vi "Database.Reload.vi"(7 "Idx":i32, 8 "error in":errorcluster, 11 "Data in":T1) -> (0 "error out":errorcluster, 3 "Data out":T1)   [LabVIEW 2016]
doc: "Connect to database\n\nWabco 2017 All right reserved\nAuthor: maciej.szupienko@wabco-auto.com"
uses:
  Database.Global.vi
  Cache/Cache.SystemID.Fglb.Action.ctl
  Cache/Cache.TestSteps.Fglb.Action.ctl
  ProdaNG/Controls/ProdaNG.TestStepParam.ctl
  ProdaNG/Controls/ProdaNG.TestValue.ctl
  ProdaNG/Controls/ProdaNG.TestStep.ctl
  Cache/Cache.TestSteps.Fglb.ResultData.ctl
  ProdaNG/Controls/ProdaNG.TestValueResult.ctl
  ProdaNG/Controls/ProdaNG.TestStepResult.ctl
  ProdaNG/Controls/ProdaNG.ProcessStepResult.ctl
  ProdaNG/Controls/ProdaNG.ProcessResult.ctl
  ProdaNG/Controls/ProdaNG.ProcessStepParam.ctl
  Cache/Cache.TestSteps.Fglb.TestData.ctl
  ProdaNG/Controls/ProdaNG.Unit.ctl
  ProdaNG/Controls/ProdaNG.Process.ctl
  ProdaNG/Controls/ProdaNG.ProcessStep.ctl
  Database.Data.Status.ctl
  Database.Data.Sets.ctl
  Database.Data.ctl
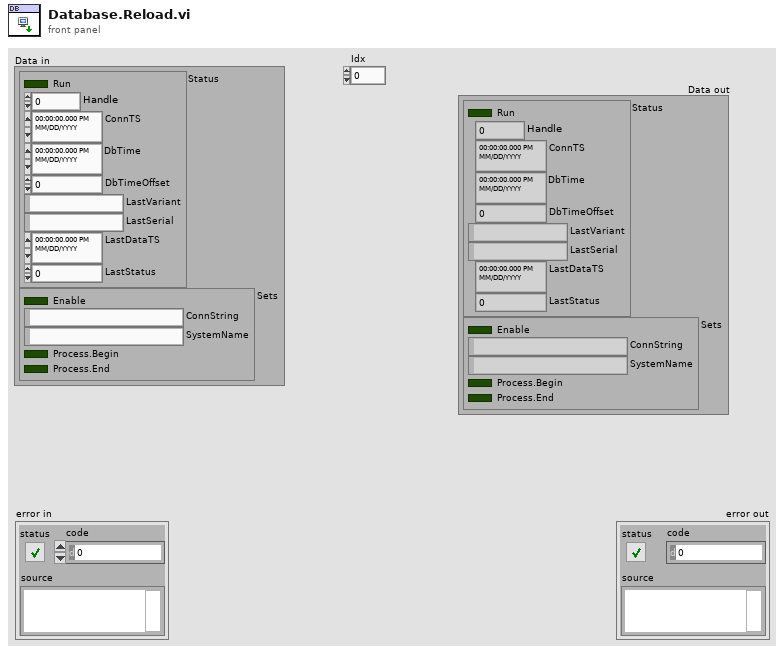
[diagram p1: front panel]
types:
  T1 = typedef "Database.Data.ctl" = cluster{"Status":T2, "Sets":T3}
  T2 = typedef "Database.Data.Status.ctl" = cluster{"Run":bool, "Handle":i32, "ConnTS":timestamp, "DbTime":timestamp, "DbTimeOffset":dbl, "LastVariant":string, "LastSerial":string, "LastDataTS":timestamp, "LastStatus":i32}
  T3 = typedef "Database.Data.Sets.ctl" = cluster{"Enable":bool, "ConnString":string, "SystemName":string, "Process.Begin":bool, "Process.End":bool}
  T4 = typedef "Cache.TestSteps.Fglb.ResultData.ctl" = cluster{"Ref":string, "Serial":string, "Pr":T5, "PSr":T6, "TSr":cluster{"TSr":T7, "TVr":T8[]}[]}
  T5 = typedef "ProdaNG.ProcessResult.ctl" = cluster{"c_id":string, "productId":string, "processId":i32, "statusId":i32, "startTime":string, "endTime":string}
  T6 = typedef "ProdaNG.ProcessStepResult.ctl" = cluster{"c_id":string, "processResultId":string, "processStepId":i32, "statusId":i32, "operatorId":i32, "startTime":string, "endTime":string}
  T7 = typedef "ProdaNG.TestStepResult.ctl" = cluster{"c_id":string, "processStepResultId":string, "testStepId":i32, "statusId":i32}
  T8 = typedef "ProdaNG.TestValueResult.ctl" = cluster{"c_id":string, "testStepResultId":string, "testValueId":i32, "result":dbl, "statusId":i32, "contentId":string}
  T9 = typedef "Cache.TestSteps.Fglb.Action.ctl" = enum16{"init", "add", "get"}
  T10 = typedef "Cache.TestSteps.Fglb.TestData.ctl" = cluster{"Ref":string, "Desc":string, "P":T11, "PS":T12, "PP":T13[], "TS":cluster{"TS":T14, "TV":T15[], "TP":T16[]}[], "Units":T17[]}
  T11 = typedef "ProdaNG.Process.ctl" = cluster{"i_id":i32, "productionLineId":i32, "releaseId":i32, "contentId":string, "previewId":string, "mdReason":string, "mdUser":string, "mdTime":string, "description":string}
  T12 = typedef "ProdaNG.ProcessStep.ctl" = cluster{"i_id":i32, "processId":i32, "systemId":i32, "releaseId":i32, "processSequence":i32, "limitYellow":dbl, "limitRed":dbl, "mdReason":string, "mdUser":string, "mdTime":string, "filename":string, "transfer":string, "description":string}
  T13 = typedef "ProdaNG.ProcessStepParam.ctl" = cluster{"i_id":i32, "processStepId":i32, "unitId":i32, "contentId":string, "previewId":string, "value":dbl, "valueText":string, "paramSequence":i32, "history":i32, "mdReason":string, "mdUser":string, "mdTime":string, "description":string}
  T14 = typedef "ProdaNG.TestStep.ctl" = cluster{"i_id":i32, "processStepId":i32, "testSequence":i32, "testOrder":i32, "mdReason":string, "mdUser":string, "mdTime":string, "description":string}
  T15 = typedef "ProdaNG.TestValue.ctl" = cluster{"i_id":i32, "testStepId":i32, "releaseId":i32, "unitId":i32, "contentId":string, "previewId":string, "maximum":dbl, "minimum":dbl, "valueText":string, "testValueSequence":i32, "history":i32, "mdReason":string, "mdUser":string, "mdTime":string, "description":string}
  T16 = typedef "ProdaNG.TestStepParam.ctl" = cluster{"i_id":i32, "testStepId":i32, "unitId":i32, "contentId":string, "previewId":string, "value":dbl, "valueText":string, "paramSequence":i32, "history":i32, "mdReason":string, "mdUser":string, "mdTime":string, "description":string}
  T17 = typedef "ProdaNG.Unit.ctl" = cluster{"i_id":i32, "name":string, "mdReason":string, "mdUser":string, "mdTime":string, "description":string}
  T18 = typedef "Cache.SystemID.Fglb.Action.ctl" = enum16{"init", "add", "get"}
  T19 = typedef "Cache.SystemID.Fglb.Action.ctl" = enum16{"init", "add", "add CheckExistSystem", "add PrevSystem", "get", "get CheckExistSystem", "get PrevSystem"}
  T20 = typedef "ProdaNG.Identification.ctl" = cluster{"processId":i32, "systemId":i32, "processStepId":i32, "wabcoPartId":i32}
  T21 = cluster{"TestStep":T14, "TestStepValues":T15[], "TestStepParams":T16[]}
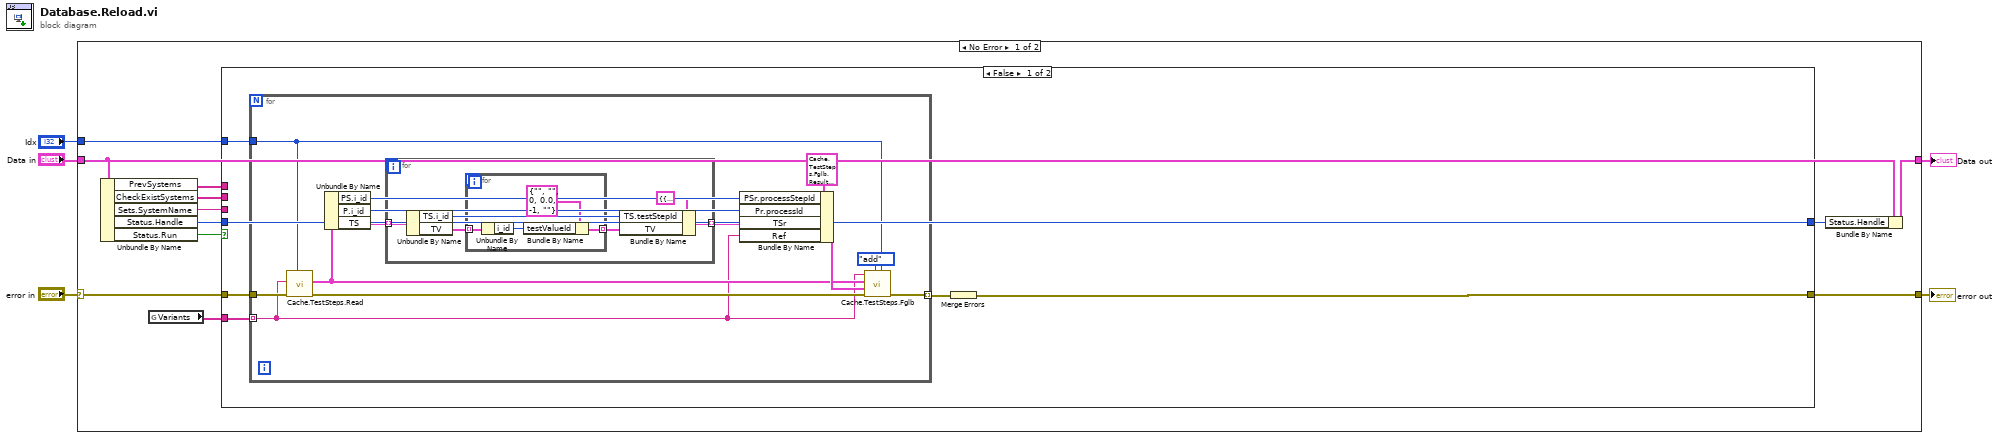
[diagram p0: block diagram]
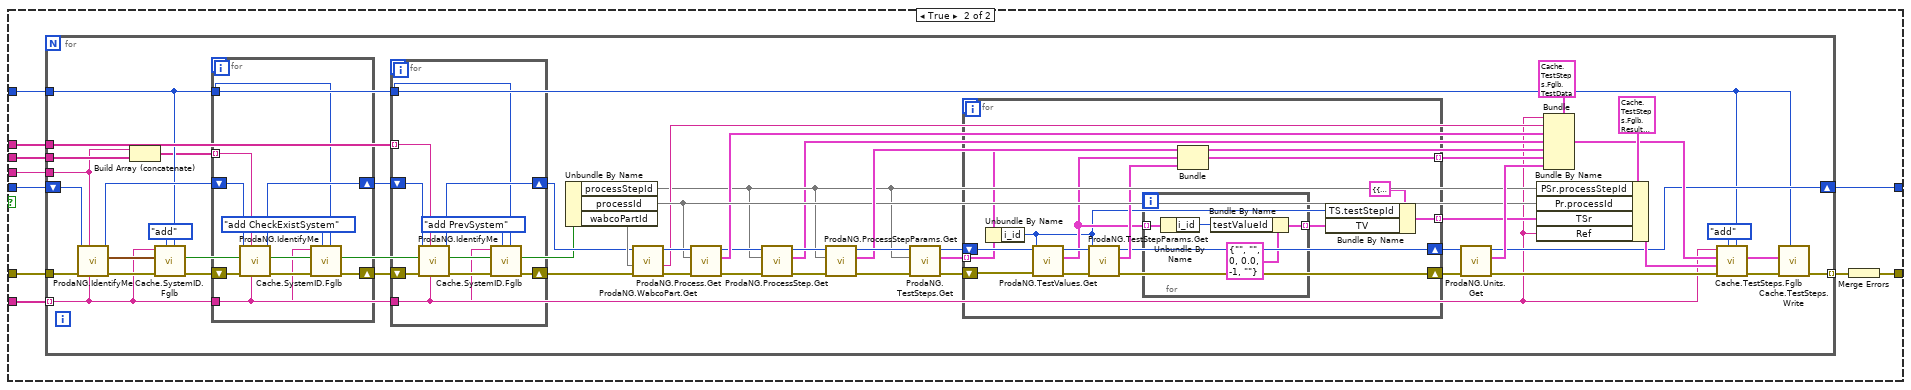
[diagram p2: hidden frame]
diagram:
  n1 = case shown="No Error" "error in" {
    selector: "error in" -> [w17 w147]
    tunnel: [w16 w147] -> w5
    tunnel: "Data in" -> [w12 w146]
    tunnel: "Idx" -> [w7 _]
    tunnel: [w10 w146] -> w1
    frame No Error {
      n2 = Unbundle By Name(w12) -> ("PrevSystems"=w15:string[], "CheckExistSystems"=w9:string[], "Sets.SystemName"=w14:string, "Status.Handle"=w13:i32, "Status.Run"=w6:bool)
      n3 = global read "Database.Global.vi" "Variants"() -> (w8:string[])
      n4 = case shown="False" w6 {
        tunnel: w17 -> [w21 w56]
        tunnel: [w18 w47] -> w16
        tunnel: w15 -> [_ w52]
        tunnel: w14 -> [_ w55]
        tunnel: w13 -> [w23 w54]
        tunnel: [w23 w49] -> w11
        tunnel: w9 -> [_ w51]
        tunnel: w8 -> [w22 w53]
        tunnel: w7 -> [w20 w48]
        frame False {
          n5 = for {
            tunnel: w22 -> [w24] mode=indexing
            tunnel: w21 -> [w36]
            tunnel: w20 -> [w31]
            tunnel: [w26] -> w19 mode=indexing
            n6 = call "Cache.TestSteps.Read.vi"("Idx"=w31, "error in (no error)"=w36, "Ref"=w24) -> ("error out"=w32:errorcluster, "TS in"=w25:T10)  [unwired: 7 in]
            n7 = Unbundle By Name(w25) -> ("PS.i_id"=w28:i32, "P.i_id"=w29:i32, "TS"=w35:cluster{"TS":T14, "TV":T15[], "TP":T16[]}[])
            n8 = for {
              tunnel: [w39] -> w27 mode=indexing
              tunnel: w35 -> [w38] mode=indexing
              n9 = Unbundle By Name(w38) -> ("TS.i_id"=w41:i32, "TV"=w37:T15[])
              n10 = for {
                tunnel: w37 -> [w46] mode=indexing
                tunnel: [w43] -> w42 mode=indexing
                n11 = Unbundle By Name(w46) -> ("i_id"=w45:i32)
                n12 = Bundle By Name(cluster=T8 {"c_id"="", "testStepResultId"="", "testValueId"=0, "result"=0.0, "statusId"=-1, "contentId"=""} ("TV"), "testValueId"=w45) -> (w43:T8)
              }
              n13 = Bundle By Name(cluster=cluster{"TS":T7, "TV":T8[]} {"TS"={"c_id"="", "processStepResultId"="", "testStepId"=0, "statusId"=-1}, "TV"=[]} ("Cluster"), "TS.testStepId"=w41, "TV"=w42) -> (w39:cluster{"TS":T7, "TV":T8[]})
            }
            n14 = Bundle By Name(cluster=T4 {"Ref"="", "Serial"="", "Pr"={"c_id"="", "productId"="", "processId"=0, "statusId"=0, "startTime"="", "endTime"=""}, "PSr"={"c_id"="", "processResultId"="", "processStepId"=0, "statusId"=0, "operatorId"=0, "startTime"="", "endTime"=""}, "TSr"=[]} ("Result in"), "PSr.processStepId"=w28, "Pr.processId"=w29, "TSr"=w27, "Ref"=w24) -> (w33:T4)
            n15 = call "Cache.TestSteps.Fglb.vi"("SystemIdx"=w31, "Action (get)"=Cache.TestSteps.Fglb.Action."add", "error in (no error)"=w32, "Result in"=w33, "Test in"=w25, "Variant"=w24) -> ("error out"=w26:errorcluster)  [unwired: 2 in, 3 out]
          }
          n16 = Merge Errors(w19) -> (w18:errorcluster)
        }
        frame True {
          n17 = for {
            tunnel: w55 -> [w58]
            tunnel: w51 -> [w104]
            shift-right: [w70] -> w49
            shift-left: w54 -> [w107]
            tunnel: w52 -> [w101]
            tunnel: w53 -> [w57] mode=indexing
            tunnel: w48 -> [w66]
            tunnel: w56 -> [w97]
            tunnel: [w68] -> w50 mode=indexing
            n18 = call "ProdaNG.IdentifyMe.vi"("wabcoNumber"=w57, "systemName"=w58, "error in"=w97, "dbHandleIn"=w107) -> ("error out"=w105:errorcluster, "Identification"=w106:T20, "dbHandle"=w103:i32)  [unwired: 5 in]
            n19 = Build Array (concatenate)(w58, w104) -> (w59:string[])
            n20 = call "Cache.SystemID.Fglb.vi"("Station"=w66, "Action (get)"=Cache.SystemID.Fglb.Action."add", "error in (no error)"=w105, "SytemID"=w106, "Variant"=w57) -> ("error out"=w100:errorcluster, "Found"=w73:bool)  [unwired: 4 in, 1 out]
            n21 = for {
              tunnel: w59 -> [w115] mode=indexing
              shift-right: [w113] -> w102
              shift-left: w103 -> [w114]
              tunnel: w57 -> [w111]
              shift-right: [w110] -> w99
              shift-left: w100 -> [w116]
              tunnel: w66 -> [w108]
              n22 = call "ProdaNG.IdentifyMe.vi"("wabcoNumber"=w111, "systemName"=w115, "error in"=w116, "dbHandleIn"=w114) -> ("error out"=w112:errorcluster, "Identification"=w117:T20, "dbHandle"=w113:i32)  [unwired: 5 in]
              n23 = call "Cache.SystemID.Fglb.vi"("Station"=w108, "Action (get)"=Cache.SystemID.Fglb.Action."add CheckExistSystem", "error in (no error)"=w112, "SytemID"=w117, "Variant"=w111) -> ("error out"=w110:errorcluster)  [unwired: 4 in, 2 out]
            }
            n24 = for {
              tunnel: w101 -> [w125] mode=indexing
              shift-right: [w123] -> w92
              shift-left: w102 -> [w124]
              tunnel: w57 -> [w121]
              shift-right: [w120] -> w93
              shift-left: w99 -> [w126]
              tunnel: w66 -> [w118]
              n25 = call "ProdaNG.IdentifyMe.vi"("wabcoNumber"=w121, "systemName"=w125, "error in"=w126, "dbHandleIn"=w124) -> ("error out"=w122:errorcluster, "Identification"=w127:T20, "dbHandle"=w123:i32)  [unwired: 5 in]
              n26 = call "Cache.SystemID.Fglb.vi"("Station"=w118, "Action (get)"=Cache.SystemID.Fglb.Action."add PrevSystem", "error in (no error)"=w122, "SytemID"=w127, "Variant"=w121) -> ("error out"=w120:errorcluster)  [unwired: 4 in, 2 out]
            }
            n27 = Unbundle By Name(w73) -> ("processStepId"=w61, "processId"=w75, "wabcoPartId"=w96)
            n28 = call "ProdaNG.WabcoPart.Get.vi"("error in (no error)"=w93, "WabcoPartId (-1: use WabcoNumber)"=w96, "dbHandleIn"=w92) -> ("error out"=w94:errorcluster, "ProductName"=w71:string, "dbHandle"=w95:i32)  [unwired: 5 in, 1 out]
            n29 = call "ProdaNG.Process.Get.vi"("error in (no error)"=w94, "processId"=w75, "dbHandleIn"=w95) -> ("error out"=w64:errorcluster, "Process"=w72:T11, "dbHandle"=w65:i32)  [unwired: 5 in, 1 out]
            n30 = call "ProdaNG.ProcessStep.Get.vi"("error in (no error)"=w64, "processStepId"=w61, "dbHandleIn"=w65) -> ("error out"=w63:errorcluster, "ProcessStep"=w60:T12, "dbHandle"=w62:i32)  [unwired: 6 in]
            n31 = call "ProdaNG.ProcessStepParams.Get.vi"("error in (no error)"=w63, "processStepId"=w61, "dbHandleIn"=w62) -> ("error out"=w90:errorcluster, "ProcStepParams"=w80:T13[], "dbHandle"=w89:i32)  [unwired: 6 in]
            n32 = call "ProdaNG.TestSteps.Get.vi"("error in (no error)"=w90, "processStepId"=w61, "dbHandleIn"=w89) -> ("error out"=w88:errorcluster, "TestSteps"=w86:T14[], "dbHandle"=w87:i32)  [unwired: 6 in]
            n33 = for {
              shift-right: [w137] -> w84
              shift-left: w88 -> [w141]
              tunnel: w86 -> [w129] mode=indexing
              tunnel: [w136] -> w85 mode=indexing
              tunnel: [w130] -> w76 mode=indexing
              shift-right: [w128] -> w83
              shift-left: w87 -> [w140]
              n34 = Unbundle By Name(w129) -> ("i_id"=w132:i32)
              n35 = call "ProdaNG.TestValues.Get.vi"("error in (no error)"=w141, "testStepId"=w132, "dbHandleIn"=w140) -> ("error out"=w138:errorcluster, "TestStepValues"=w133:T15[], "dbHandle"=w139:i32)  [unwired: 6 in]
              n36 = call "ProdaNG.TestStepParams.Get.vi"("error in (no error)"=w138, "testStepId"=w132, "dbHandleIn"=w139) -> ("error out"=w137:errorcluster, "TestStepParams"=w135:T16[], "dbHandle"=w128:i32)  [unwired: 6 in]
              n37 = for {
                tunnel: w133 -> [w145] mode=indexing
                tunnel: [w142] -> w134 mode=indexing
                n38 = Unbundle By Name(w145) -> ("i_id"=w144:i32)
                n39 = Bundle By Name(cluster=T8 {"c_id"="", "testStepResultId"="", "testValueId"=0, "result"=0.0, "statusId"=-1, "contentId"=""} ("TV"), "testValueId"=w144) -> (w142:T8)
              }
              n40 = Bundle("TestStep"=w129, "TestStepValues"=w133, "TestStepParams"=w135) -> (w136:T21)  [unwired: 1 in]
              n41 = Bundle By Name(cluster=cluster{"TS":T7, "TV":T8[]} {"TS"={"c_id"="", "processStepResultId"="", "testStepId"=0, "statusId"=-1}, "TV"=[]} ("Cluster"), "TS.testStepId"=w132, "TV"=w134) -> (w130:cluster{"TS":T7, "TV":T8[]})
            }
            n42 = call "ProdaNG.Units.Get.vi"("error in (no error)"=w84, "dbHandleIn"=w83) -> ("error out"=w77:errorcluster, "units"=w82:T17[], "dbHandle"=w70:i32)  [unwired: 6 in, 1 out]
            n43 = Bundle By Name(cluster=T4 {"Ref"="", "Serial"="", "Pr"={"c_id"="", "productId"="", "processId"=0, "statusId"=0, "startTime"="", "endTime"=""}, "PSr"={"c_id"="", "processResultId"="", "processStepId"=0, "statusId"=0, "operatorId"=0, "startTime"="", "endTime"=""}, "TSr"=[]} ("Result in"), "PSr.processStepId"=w61, "Pr.processId"=w75, "TSr"=w76, "Ref"=w57) -> (w78:T4)
            n44 = Bundle(cluster=T10 {"Ref"="", "Desc"="", "P"={"i_id"=0, "productionLineId"=0, "releaseId"=0, "contentId"="", "previewId"="", "mdReason"="", "mdUser"="", "mdTime"="", "description"=""}, "PS"={"i_id"=0, "processId"=0, "systemId"=0, "releaseId"=0, "processSequence"=0, "limitYellow"=0.0, "limitRed"=0.0, "mdReason"="", "mdUser"="", "mdTime"="", "filename"="", "transfer"="", "description"=""}, "PP"=[], "TS"=[], "Units"=[]} ("TestStep in"), "Ref"=w57, "Desc"=w71, "P"=w72, "PS"=w60, "PP"=w80, "TS"=w85, "Units"=w82) -> (w74:T10)
            n45 = call "Cache.TestSteps.Fglb.vi"("SystemIdx"=w66, "Action (get)"=Cache.TestSteps.Fglb.Action."add", "error in (no error)"=w77, "Result in"=w78, "Test in"=w74, "Variant"=w57) -> ("error out"=w69:errorcluster, "Test out"=w67:T10)  [unwired: 2 in, 2 out]
            n46 = call "Cache.TestSteps.Write.vi"("Idx"=w66, "error in (no error)"=w69, "TS in"=w67) -> ("error out"=w68:errorcluster)  [unwired: 8 in]
          }
          n47 = Merge Errors(w50) -> (w47:errorcluster)
        }
      }
      n48 = Bundle By Name(cluster=w12, "Status.Handle"=w11) -> (w10:T1)
    }
    frame Error {
    }
  }
  "error out" <- w5
  "Data out" <- w1
